vi "确定测试初始化（测试软件版本，说明书版本）.vi"(1 "测试说明界面参数输入":T1, 2 "说明书版本":string, 3 "测试软件":string) -> (0 "测试说明界面参数输出":T1)   [LabVIEW 2015]
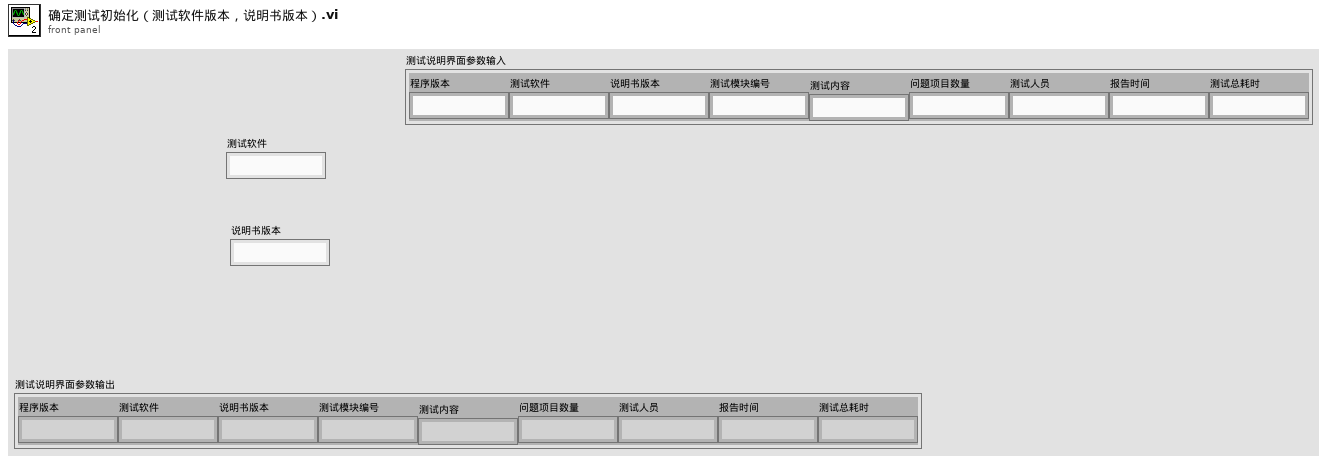
[diagram p1: front panel]
types:
  T1 = typedef "测试说明界面参数.ctl" = cluster{"程序版本":string, "测试软件":string, "说明书版本":string, "测试模块编号":string, "测试内容":string, "问题项目数量":string, "测试人员":string, "报告时间":string, "测试总耗时":string}
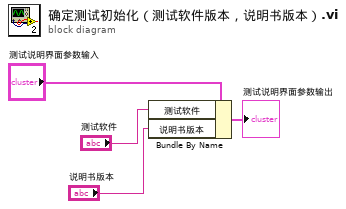
[diagram p0: block diagram]
diagram:
  n1 = Bundle By Name(cluster="测试说明界面参数输入", "测试软件"="测试软件", "说明书版本"="说明书版本") -> (→"测试说明界面参数输出":T1)
